vi "jog_motors.vi"(0 "up 2":bool, 1 "up 4":bool, 2 "up 5":bool, 3 "Numeric 2":dbl, 4 "Numeric 4":dbl, 5 "down 2":bool, 7 "Numeric":dbl, 9 "up 3":bool, 11 "down 3":bool, 12 "down 4":bool, 13 "down 5":bool, 14 "Numeric 3":dbl) -> (6 "increment":dbl=1.0)   [LabVIEW 2025]
uses:
  increment_global_var.vi
panel:
  in  "stop":bool
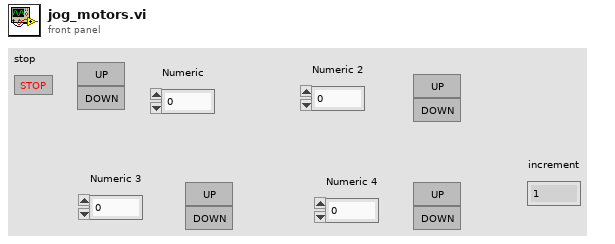
[diagram p1: front panel]
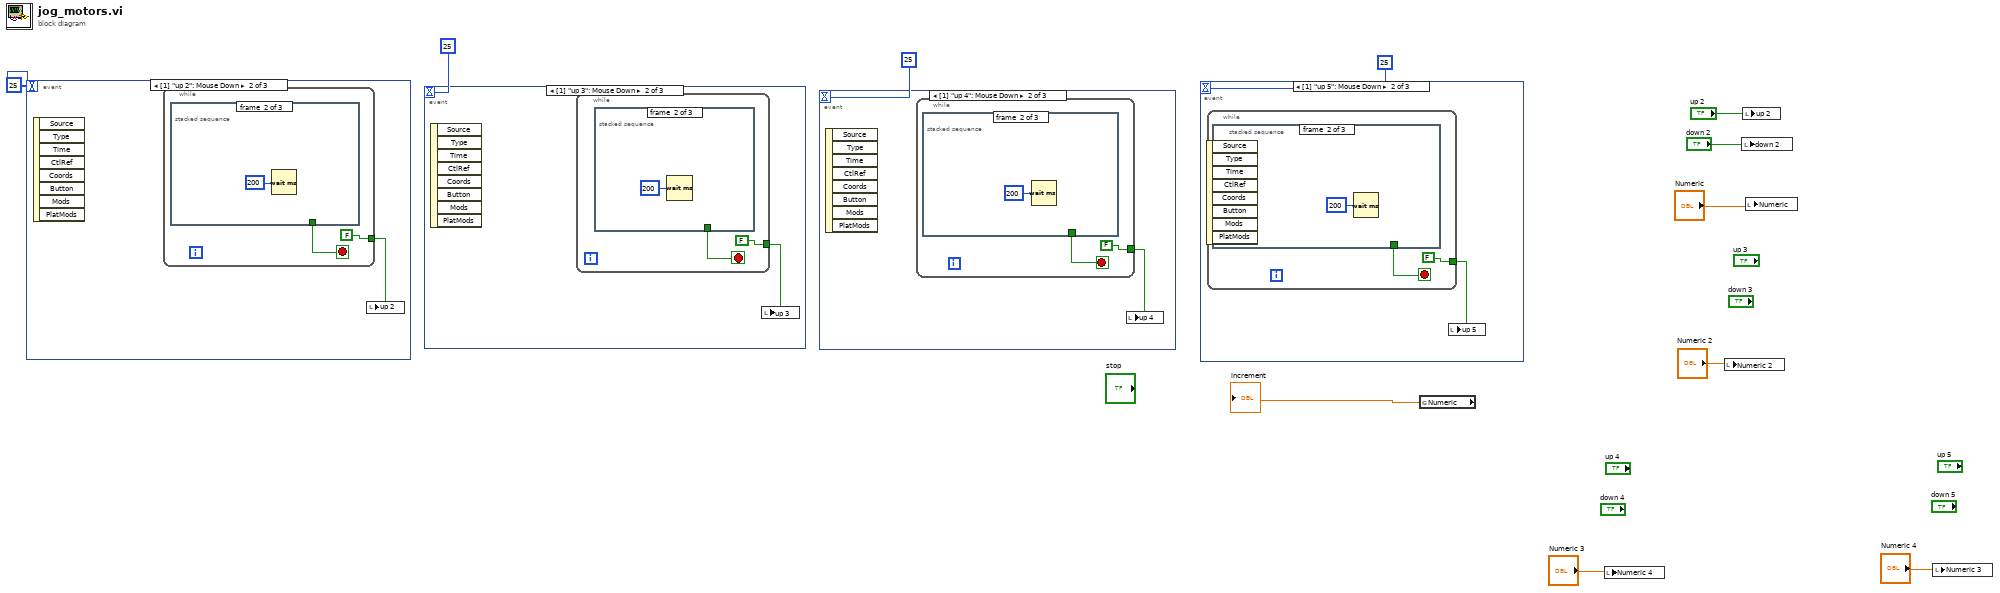
[diagram p0: block diagram]
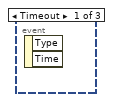
[diagram p2: hidden frame]
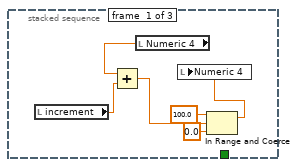
[diagram p3: hidden frame]
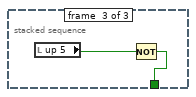
[diagram p4: hidden frame]
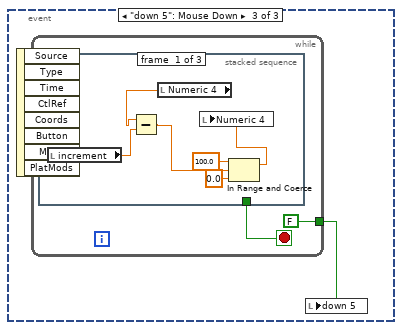
[diagram p5: hidden frame]
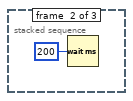
[diagram p6: hidden frame]
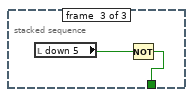
[diagram p7: hidden frame]
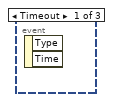
[diagram p8: hidden frame]
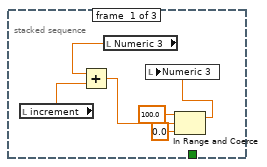
[diagram p9: hidden frame]
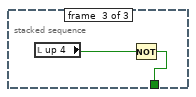
[diagram p10: hidden frame]
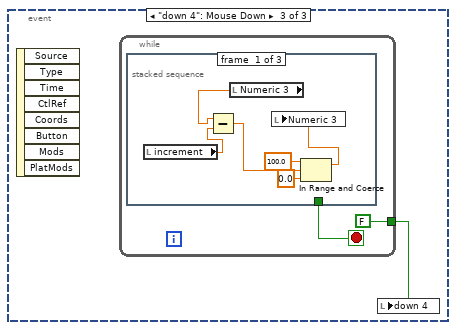
[diagram p11: hidden frame]
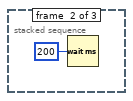
[diagram p12: hidden frame]
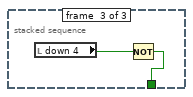
[diagram p13: hidden frame]
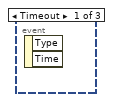
[diagram p14: hidden frame]
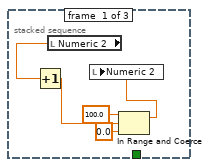
[diagram p15: hidden frame]
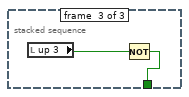
[diagram p16: hidden frame]
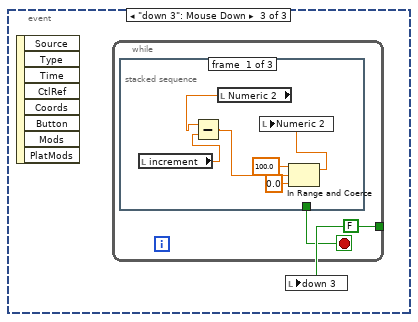
[diagram p17: hidden frame]
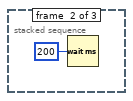
[diagram p18: hidden frame]
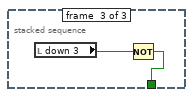
[diagram p19: hidden frame]
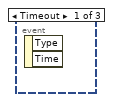
[diagram p20: hidden frame]
diagram:
  n1 = event shown="[1] \"up 2\": Mouse Down" {
    selector: _ -> [_ _ _]
    dyn-events: _ -> [_ _ _]
    timeout: 25 -> [_ _ _]
    event Timeout {
      n2 = event-data() -> ()  [unwired: 1 in, 2 out]
    }
    event "up 2": Mouse Down {
      n3 = event-data() -> ()  [unwired: 1 in, 8 out]
      n4 = while {
        tunnel: [FALSE] -> w12
        stop <- w14 stop-if-true
        n5 = stacked-sequence {
          tunnel: [_ _ w23] -> w14
          frame #0 {
            n6 = local read "increment"() -> (w15:dbl)
            n7 = local read "Numeric"() -> (w16:dbl)
            n8 = Add(x=w16, y=w15) -> (x+y=w17:dbl)
            n9 = In Range and Coerce(upper limit=100.0 ("oberer Grenzwert"), x=w17, lower limit=0.0 ("unterer Grenzwert")) -> (coerced(x)=w18:dbl)  [unwired: 1 out]
            n10 = local write "Numeric"(w18) -> ()
          }
          frame #1 {
            n11 = Wait (ms)(milliseconds to wait=u32 200 ("Zu wartende ms")) -> ()  [unwired: 1 out]
          }
          frame #2 {
            n12 = local read "up 2"() -> (w22:bool)
            n13 = Not(x=w22) -> (.not. x?=w23:bool)
          }
        }
      }
      n14 = local write "up 2"(w12) -> ()
    }
    event "down 2": Mouse Down {
      n15 = event-data() -> ()  [unwired: 1 in, 8 out]
      n16 = while {
        tunnel: [FALSE] -> w24
        stop <- w26 stop-if-true
        n17 = stacked-sequence {
          tunnel: [_ _ w35] -> w26
          frame #0 {
            n18 = local read "increment"() -> (w27:dbl)
            n19 = local read "Numeric"() -> (w28:dbl)
            n20 = Subtract(x=w28, y=w27) -> (x-y=w29:dbl)
            n21 = In Range and Coerce(upper limit=100.0 ("oberer Grenzwert"), x=w29, lower limit=0.0 ("unterer Grenzwert")) -> (coerced(x)=w30:dbl)  [unwired: 1 out]
            n22 = local write "Numeric"(w30) -> ()
          }
          frame #1 {
            n23 = Wait (ms)(milliseconds to wait=u32 200 ("Zu wartende ms")) -> ()  [unwired: 1 out]
          }
          frame #2 {
            n24 = local read "down 2"() -> (w34:bool)
            n25 = Not(x=w34) -> (.not. x?=w35:bool)
          }
        }
      }
      n26 = local write "down 2"(w24) -> ()
    }
  }
  n27 = event shown="[1] \"up 3\": Mouse Down" {
    selector: _ -> [_ _ _]
    dyn-events: _ -> [_ _ _]
    timeout: 25 -> [_ _ _]
    event Timeout {
      n28 = event-data() -> ()  [unwired: 1 in, 2 out]
    }
    event "up 3": Mouse Down {
      n29 = event-data() -> ()  [unwired: 1 in, 8 out]
      n30 = while {
        tunnel: [FALSE] -> w36
        stop <- w38 stop-if-true
        n31 = stacked-sequence {
          tunnel: [_ _ w46] -> w38
          frame #0 {
            n32 = local read "Numeric 2"() -> (w43:dbl)
            n33 = Increment(x=w43) -> (x+1=w42:dbl)
            n34 = In Range and Coerce(upper limit=100.0 ("oberer Grenzwert"), x=w42, lower limit=0.0 ("unterer Grenzwert")) -> (coerced(x)=w39:dbl)  [unwired: 1 out]
            n35 = local write "Numeric 2"(w39) -> ()
          }
          frame #1 {
            n36 = Wait (ms)(milliseconds to wait=u32 200 ("Zu wartende ms")) -> ()  [unwired: 1 out]
          }
          frame #2 {
            n37 = local read "up 3"() -> (w45:bool)
            n38 = Not(x=w45) -> (.not. x?=w46:bool)
          }
        }
      }
      n39 = local write "up 3"(w36) -> ()
    }
    event "down 3": Mouse Down {
      n40 = event-data() -> ()  [unwired: 1 in, 8 out]
      n41 = while {
        tunnel: [FALSE] -> w47
        stop <- w49 stop-if-true
        n42 = stacked-sequence {
          tunnel: [_ _ w58] -> w49
          frame #0 {
            n43 = local read "increment"() -> (w50:dbl)
            n44 = local read "Numeric 2"() -> (w51:dbl)
            n45 = Subtract(x=w51, y=w50) -> (x-y=w52:dbl)
            n46 = In Range and Coerce(upper limit=100.0 ("oberer Grenzwert"), x=w52, lower limit=0.0 ("unterer Grenzwert")) -> (coerced(x)=w53:dbl)  [unwired: 1 out]
            n47 = local write "Numeric 2"(w53) -> ()
          }
          frame #1 {
            n48 = Wait (ms)(milliseconds to wait=u32 200 ("Zu wartende ms")) -> ()  [unwired: 1 out]
          }
          frame #2 {
            n49 = local read "down 3"() -> (w57:bool)
            n50 = Not(x=w57) -> (.not. x?=w58:bool)
          }
        }
      }
      n51 = local write "down 3"(w47) -> ()
    }
  }
  n52 = event shown="[1] \"up 4\": Mouse Down" {
    selector: _ -> [_ _ _]
    dyn-events: _ -> [_ _ _]
    timeout: 25 -> [_ _ _]
    event Timeout {
      n53 = event-data() -> ()  [unwired: 1 in, 2 out]
    }
    event "up 4": Mouse Down {
      n54 = event-data() -> ()  [unwired: 1 in, 8 out]
      n55 = while {
        tunnel: [FALSE] -> w59
        stop <- w61 stop-if-true
        n56 = stacked-sequence {
          tunnel: [_ _ w70] -> w61
          frame #0 {
            n57 = local read "increment"() -> (w63:dbl)
            n58 = local read "Numeric 3"() -> (w62:dbl)
            n59 = Add(x=w62, y=w63) -> (x+y=w64:dbl)
            n60 = In Range and Coerce(upper limit=100.0 ("oberer Grenzwert"), x=w64, lower limit=0.0 ("unterer Grenzwert")) -> (coerced(x)=w65:dbl)  [unwired: 1 out]
            n61 = local write "Numeric 3"(w65) -> ()
          }
          frame #1 {
            n62 = Wait (ms)(milliseconds to wait=u32 200 ("Zu wartende ms")) -> ()  [unwired: 1 out]
          }
          frame #2 {
            n63 = local read "up 4"() -> (w69:bool)
            n64 = Not(x=w69) -> (.not. x?=w70:bool)
          }
        }
      }
      n65 = local write "up 4"(w59) -> ()
    }
    event "down 4": Mouse Down {
      n66 = event-data() -> ()  [unwired: 1 in, 8 out]
      n67 = while {
        tunnel: [FALSE] -> w71
        stop <- w73 stop-if-true
        n68 = stacked-sequence {
          tunnel: [_ _ w82] -> w73
          frame #0 {
            n69 = local read "increment"() -> (w74:dbl)
            n70 = local read "Numeric 3"() -> (w75:dbl)
            n71 = Subtract(x=w75, y=w74) -> (x-y=w76:dbl)
            n72 = In Range and Coerce(upper limit=100.0 ("oberer Grenzwert"), x=w76, lower limit=0.0 ("unterer Grenzwert")) -> (coerced(x)=w77:dbl)  [unwired: 1 out]
            n73 = local write "Numeric 3"(w77) -> ()
          }
          frame #1 {
            n74 = Wait (ms)(milliseconds to wait=u32 200 ("Zu wartende ms")) -> ()  [unwired: 1 out]
          }
          frame #2 {
            n75 = local read "down 4"() -> (w81:bool)
            n76 = Not(x=w81) -> (.not. x?=w82:bool)
          }
        }
      }
      n77 = local write "down 4"(w71) -> ()
    }
  }
  n78 = event shown="[1] \"up 5\": Mouse Down" {
    selector: _ -> [_ _ _]
    dyn-events: _ -> [_ _ _]
    timeout: 25 -> [_ _ _]
    event Timeout {
      n79 = event-data() -> ()  [unwired: 1 in, 2 out]
    }
    event "up 5": Mouse Down {
      n80 = event-data() -> ()  [unwired: 1 in, 8 out]
      n81 = while {
        tunnel: [FALSE] -> w83
        stop <- w85 stop-if-true
        n82 = stacked-sequence {
          tunnel: [_ _ w94] -> w85
          frame #0 {
            n83 = local read "increment"() -> (w86:dbl)
            n84 = local read "Numeric 4"() -> (w87:dbl)
            n85 = Add(x=w87, y=w86) -> (x+y=w88:dbl)
            n86 = In Range and Coerce(upper limit=100.0 ("oberer Grenzwert"), x=w88, lower limit=0.0 ("unterer Grenzwert")) -> (coerced(x)=w89:dbl)  [unwired: 1 out]
            n87 = local write "Numeric 4"(w89) -> ()
          }
          frame #1 {
            n88 = Wait (ms)(milliseconds to wait=u32 200 ("Zu wartende ms")) -> ()  [unwired: 1 out]
          }
          frame #2 {
            n89 = local read "up 5"() -> (w93:bool)
            n90 = Not(x=w93) -> (.not. x?=w94:bool)
          }
        }
      }
      n91 = local write "up 5"(w83) -> ()
    }
    event "down 5": Mouse Down {
      n92 = event-data() -> ()  [unwired: 1 in, 8 out]
      n93 = while {
        tunnel: [FALSE] -> w95
        stop <- w97 stop-if-true
        n94 = stacked-sequence {
          tunnel: [_ _ w106] -> w97
          frame #0 {
            n95 = local read "increment"() -> (w98:dbl)
            n96 = local read "Numeric 4"() -> (w99:dbl)
            n97 = Subtract(x=w99, y=w98) -> (x-y=w100:dbl)
            n98 = In Range and Coerce(upper limit=100.0 ("oberer Grenzwert"), x=w100, lower limit=0.0 ("unterer Grenzwert")) -> (coerced(x)=w101:dbl)  [unwired: 1 out]
            n99 = local write "Numeric 4"(w101) -> ()
          }
          frame #1 {
            n100 = Wait (ms)(milliseconds to wait=u32 200 ("Zu wartende ms")) -> ()  [unwired: 1 out]
          }
          frame #2 {
            n101 = local read "down 5"() -> (w105:bool)
            n102 = Not(x=w105) -> (.not. x?=w106:bool)
          }
        }
      }
      n103 = local write "down 5"(w95) -> ()
    }
  }
  n104 = global read "increment_global_var.vi" "Numeric"() -> (→"increment":dbl)
  n105 = local write "Numeric 4"("Numeric 3") -> ()
  n106 = local write "Numeric 2"("Numeric 2") -> ()
  n107 = local write "down 2"("down 2") -> ()
  n108 = local write "up 2"("up 2") -> ()
  n109 = local write "Numeric"("Numeric") -> ()
  n110 = local write "Numeric 3"("Numeric 4") -> ()
